vi "TestLineto.vi"(8 "error in (no error)":errorcluster) -> (0 "error out":errorcluster)   [LabVIEW 2019]
uses:
  PathCommands.LineTo/PathCommands.LineTo.lvclass
  <vilib>/addons/_JKI Toolkits/Caraya/classes/Assert/Assert True.vi
  <vilib>/addons/_JKI Toolkits/Caraya/classes/Assert/Assert False.vi
  <vilib>/addons/_JKI Toolkits/Caraya/classes/Assert/Assert Equal Value_Variant.vi
  <vilib>/addons/_JKI Toolkits/Caraya/classes/Test/Test.lvclass
  <vilib>/addons/_JKI Toolkits/Caraya/classes/Assert/Assert.lvclass
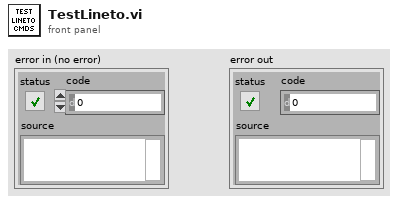
[diagram p1: front panel]
types:
  T1 = enum16{"None", "After", "Before", "Last", "First"}[]
  T2 = typedef "PathCommands.lvclass/Point.ctl" = cluster{"X":dbl, "Y":dbl}
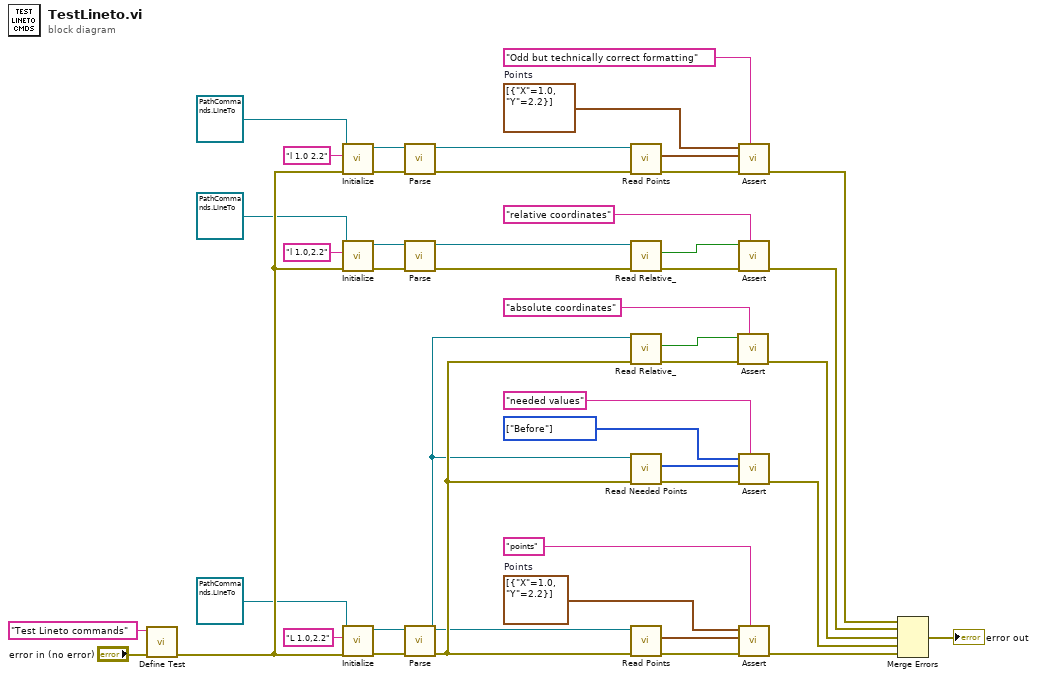
[diagram p0: block diagram]
diagram:
  w8 = cluster{"X":dbl, "Y":dbl}[] [{"X"=1.0, "Y"=2.2}]  # Points
  w29 = T1 [enum."Before"] items=["None", "After", "Before", "Last", "First"] ("Needed Points 4")
  w26 = cluster{"X":dbl, "Y":dbl}[] [{"X"=1.0, "Y"=2.2}]  # Points
  n1 = call <vilib>:"Define Test.vi"("error in (no error)"="error in (no error)", "Label (VI Title)"="Test Lineto commands") -> ("error out"=w14:errorcluster)  [unwired: 8 in, 1 out]
  n2 = call-dynamic "Initialize.vi"("error in (no error)"=w14, "CommandText"="l 1.0 2.2", "PathCommands.LineTo in"=refnum<class "PathCommands.LineTo.lvclass"> refnum ("PathCommands.LineTo.lvclass")) -> ("error out"=w17:errorcluster, "PathCommands.LineTo out"=w15:refnum<class "PathCommands.LineTo.lvclass">)  [unwired: 7 in]
  n3 = call-dynamic "Initialize.vi"("error in (no error)"=w14, "CommandText"="l 1.0,2.2", "PathCommands.LineTo in"=refnum<class "PathCommands.LineTo.lvclass"> refnum ("PathCommands.LineTo.lvclass")) -> ("error out"=w37:errorcluster, "PathCommands.LineTo out"=w39:refnum<class "PathCommands.LineTo.lvclass">)  [unwired: 7 in]
  n4 = call-dynamic "Initialize.vi"("error in (no error)"=w14, "CommandText"="L 1.0,2.2", "PathCommands.LineTo in"=refnum<class "PathCommands.LineTo.lvclass"> refnum ("PathCommands.LineTo.lvclass")) -> ("error out"=w20:errorcluster, "PathCommands.LineTo out"=w18:refnum<class "PathCommands.LineTo.lvclass">)  [unwired: 7 in]
  n5 = call-dynamic "Parse.vi"("error in (no error)"=w17, "PathCommands.LineTo in"=w15) -> ("error out"=w11:errorcluster, "PathCommands.LineTo out"=w12:refnum<class "PathCommands.LineTo.lvclass">)  [unwired: 8 in]
  n6 = call-dynamic "Parse.vi"("error in (no error)"=w37, "PathCommands.LineTo in"=w39) -> ("error out"=w43:errorcluster, "PathCommands.LineTo out"=w44:refnum<class "PathCommands.LineTo.lvclass">)  [unwired: 8 in]
  n7 = call-dynamic "Parse.vi"("error in (no error)"=w20, "PathCommands.LineTo in"=w18) -> ("error out"=w34:errorcluster, "PathCommands.LineTo out"=w31:refnum<class "PathCommands.LineTo.lvclass">)  [unwired: 8 in]
  n8 = call-dynamic "Read Points.vi"("error in (no error)"=w11, "PathCommands in"=w12) -> ("error out"=w10:errorcluster, "Points"=w9:T2[])  [unwired: 7 in, 1 out]
  n9 = call-dynamic "Read Relative_.vi"("error in (no error)"=w43, "PathCommands in"=w44) -> ("error out"=w41:errorcluster, "Relative?"=w42:bool)  [unwired: 7 in, 1 out]
  n10 = call-dynamic "Read Relative_.vi"("error in (no error)"=w34, "PathCommands in"=w31) -> ("error out"=w33:errorcluster, "Relative?"=w32:bool)  [unwired: 7 in, 1 out]
  n11 = call-dynamic "Read Needed Points.vi"("error in (no error)"=w34, "PathCommands in"=w31) -> ("error out"=w28:errorcluster, "Needed Points"=w27:T1)  [unwired: 7 in, 1 out]
  n12 = call-dynamic "Read Points.vi"("error in (no error)"=w34, "PathCommands in"=w31) -> ("error out"=w24:errorcluster, "Points"=w25:T2[])  [unwired: 7 in, 1 out]
  n13 = call-poly <vilib>:"Assert.vi"("Label"="absolute coordinates", "error in (no error)"=w33, "False?"=w32) -> ("error out"=w6:errorcluster)  [unwired: 7 in, 1 out]
  n14 = call-poly <vilib>:"Assert.vi"("Label"="Odd but technically correct formatting", "error in (no error)"=w10, "Y"=w9, "X"=w8) -> ("error out"=w4:errorcluster)  [unwired: 6 in, 1 out]
  n15 = call-poly <vilib>:"Assert.vi"("Label"="relative coordinates", "error in (no error)"=w41, "True?"=w42) -> ("error out"=w5:errorcluster)  [unwired: 7 in, 1 out]
  n16 = call-poly <vilib>:"Assert.vi"("Label"="needed values", "error in (no error)"=w28, "Y"=w27, "X"=w29) -> ("error out"=w7:errorcluster)  [unwired: 6 in, 1 out]
  n17 = call-poly <vilib>:"Assert.vi"("Label"="points", "error in (no error)"=w24, "Y"=w25, "X"=w26) -> ("error out"=w21:errorcluster)  [unwired: 6 in, 1 out]
  n18 = Merge Errors(w4, w5, w6, w7, w21) -> (→"error out":errorcluster)
